vi "Practica02.vi"() -> ()   [LabVIEW 2020]
uses:
  <vilib>/express/express shared/transition.llb/Dynamic To Waveform Array.vi
  <vilib>/express/express signal manip/GetorSetDDTAttributes/Set DDT Attributes/SetT0.vi
  <vilib>/express/express shared/transition.llb/Waveform Array To Dynamic.vi
  <vilib>/express/express signal manip/GetorSetDDTAttributes/Set DDT Attributes/Set DDT Properties.xnode
panel:
  out "Lectura":dbl
  in  "Valor máximo":dbl=70.0
  in  "Valor mínimo":dbl
  in  "Habilitar almacenamiento de datos":bool=TRUE caption="Flush? (T)"
  out "Valor dentro de rango":bool
  in  "stop":bool
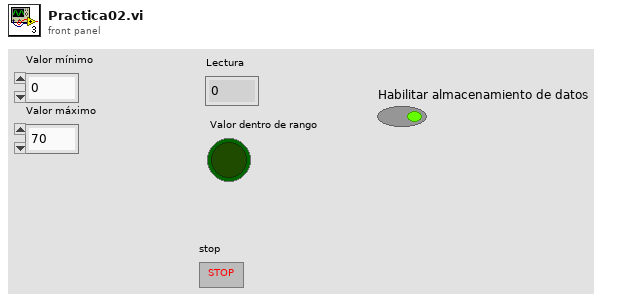
[diagram p1: front panel]
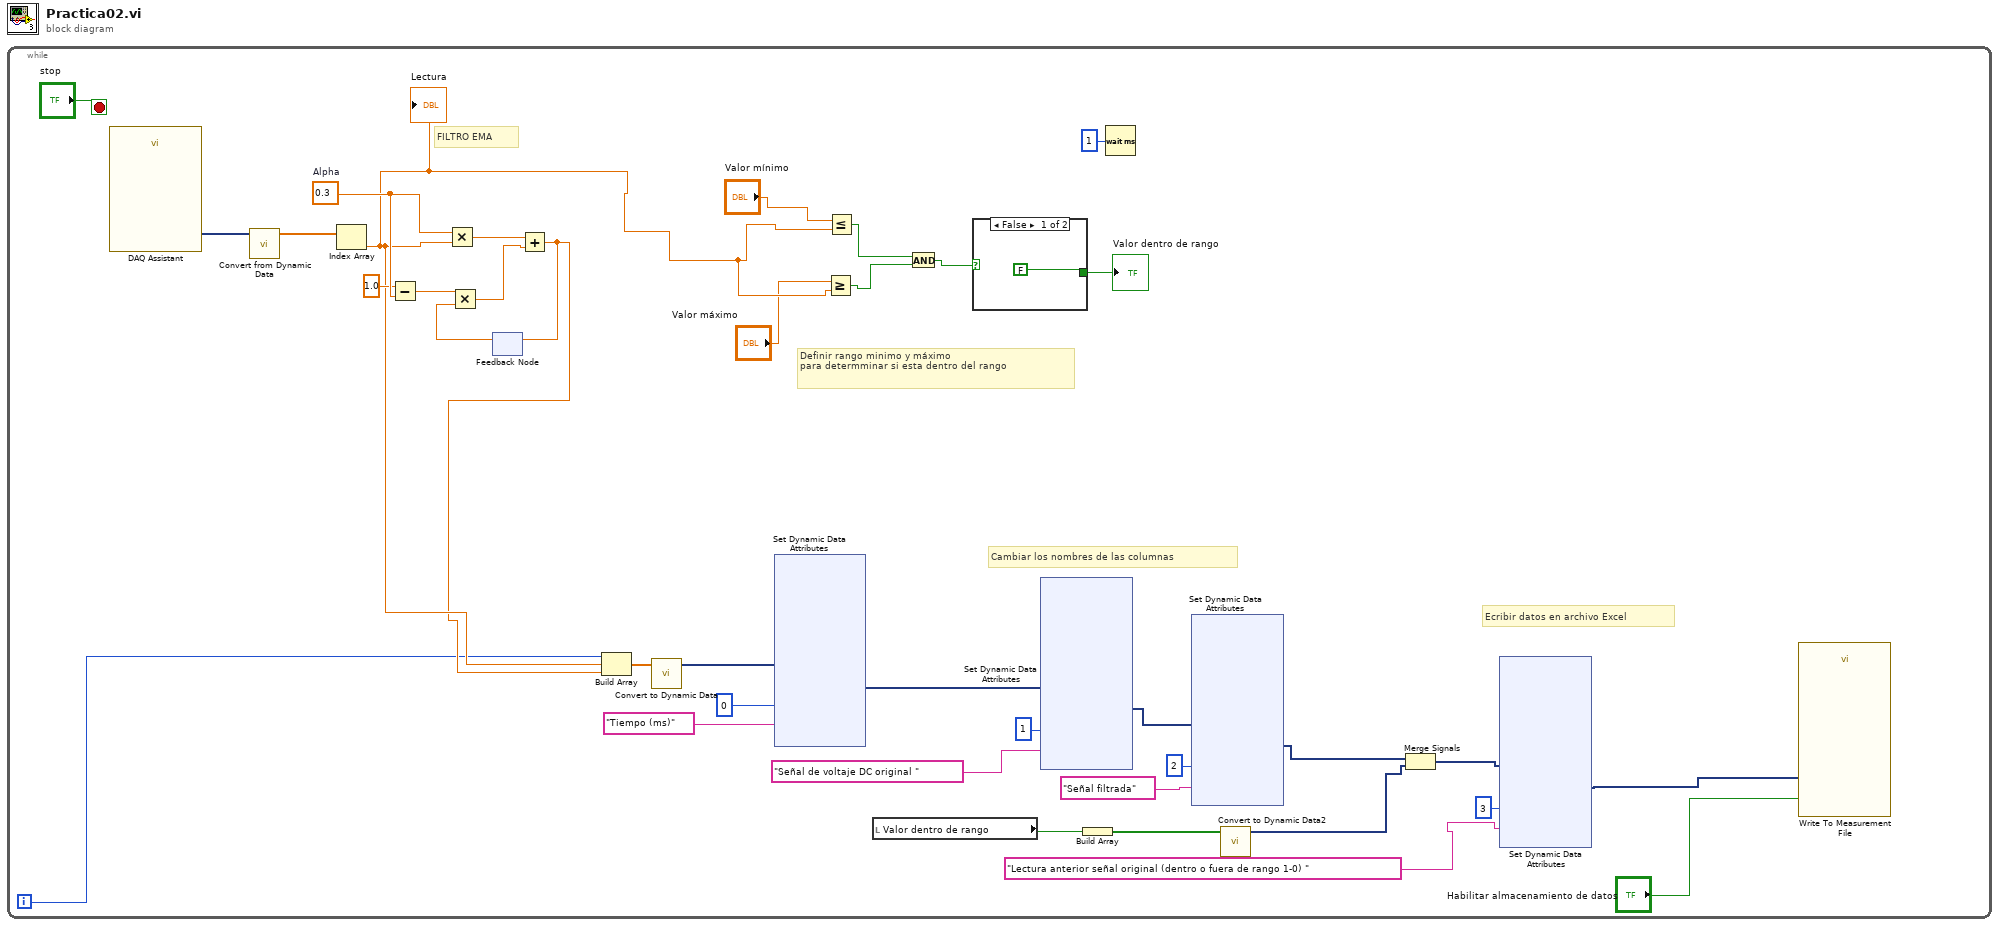
[diagram p0: block diagram]
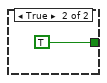
[diagram p2: hidden frame]
diagram:
  n1 = while {
    i -> [w4]
    stop <- "stop" stop-if-true
    w36 = 0.3  # Alpha
    # "Ecribir datos en archivo Excel"
    # "Cambiar los nombres de las columnas"
    # "Definir rango minimo y máximo\npara determminar si esta dentro del rango"
    # "FILTRO EMA"
    n2 = call "DAQ Assistant"() -> ("data"=w32:dynamicdata)  [unwired: 17 in, 2 out]
    n3 = call "Convert from Dynamic Data"("Dynamic Data Type"=w32) -> ("Array"=w31:dbl[])  [unwired: 3 in]
    n4 = Index Array "Index Array"(array=w31) -> (element=w6:dbl)  [unwired: 1 in]
    "Lectura" <- w6
    n5 = Subtract(x=1.0, y=w36) -> (x-y=w37:dbl)
    n6 = Multiply(x=w36, y=w6) -> (x*y=w34:dbl)
    n7 = feedback #1() -> (w38:dbl)  [unwired: 1 in]
    n8 = Multiply(x=w37, y=w38) -> (x*y=w33:dbl)
    n9 = Add(x=w34, y=w33) -> (x+y=w5:dbl)
    n10 = feedback-in #1(w5) -> ()
    n11 = Build Array(w4, w6, w5) -> (w17:dbl[])
    n12 = call "Convert to Dynamic Data"("Array"=w17) -> ("Dynamic Data Type"=w15:dynamicdata)  [unwired: 3 in]
    n13 = xnode "Set Dynamic Data Attributes"("Signals In"=w15, "Signal Index"=0, "Signal Name"="Tiempo (ms)") -> ("Signals Out"=w16:dynamicdata)  [unwired: 1 in, 1 out]
    n14 = Greater Or Equal?(x="Valor máximo", y=w6) -> (x >= y?=w26:bool)
    n15 = Less Or Equal?(x="Valor mínimo", y=w6) -> (x <= y?=w27:bool)
    n16 = local read "Valor dentro de rango"() -> (w18:bool)
    n17 = And(x=w27, y=w26) -> (x .and. y?=w28:bool)
    n18 = case shown="False" w28 {
      tunnel: [FALSE TRUE] -> w29
      frame False {
      }
      frame True {
      }
    }
    "Valor dentro de rango" <- w29
    n19 = xnode "Set Dynamic Data Attributes"("Signals In"=w16, "Signal Index"=1, "Signal Name"="Señal de voltaje DC original ") -> ("Signals Out"=w23:dynamicdata)  [unwired: 1 in, 1 out]
    n20 = Build Array(w18) -> (w19:bool[])
    n21 = Wait (ms)(milliseconds to wait=u32 1) -> ()  [unwired: 1 out]
    n22 = xnode "Set Dynamic Data Attributes"("Signals In"=w23, "Signal Index"=2, "Signal Name"="Señal filtrada") -> ("Signals Out"=w21:dynamicdata)  [unwired: 1 in, 1 out]
    n23 = call "Convert to Dynamic Data2"("Array"=w19) -> ("Dynamic Data Type"=w20:dynamicdata)  [unwired: 3 in]
    n24 = Merge Signals(w21, w20) -> (w10:dynamicdata)
    n25 = xnode "Set Dynamic Data Attributes"("Signals In"=w10, "Signal Index"=3, "Signal Name"="Lectura anterior señal original (dentro o fuera de rango 1-0) ") -> ("Signals Out"=w12:dynamicdata)  [unwired: 1 in, 1 out]
    n26 = call "Write To Measurement File"("Signals"=w12, "Flush? (T)"="Habilitar almacenamiento de datos") -> ()  [unwired: 15 in, 3 out]
  }
